vi "WS1021 CP Setting.vi"(4 "Manual Setting":i32(ring) items=["CP OFF", "CP ON", "OTP OFF", "CP 24V", "CP 26V", "CP 28V", "CP 30V", "CP 31V", "CP 32V", "CP 33V", "CP 34V", "CP 35V", "CP 36V", "CP 37V", "CP 38V", "CP 39V", "CP 40V", "CP 41V", "CP 42V", "CP 43V", "CP 44V", "CP 45V", "CP 46V", "CP 47V", "CP 48V", "CP 49V", "CP 50V", "CP 51V", "CP 52V", "CP 53V", "CP 54V", "CP 56V", "CP 58V", "CP 60V", "CP 62V"], 6 "FPGA":T1, 8 "Error In":errorcluster) -> (0 "Error Out":errorcluster, 3 "CP Select":string)   [LabVIEW 2017]
uses:
  WS_VCAP Driver 039/Source/WSVCAP Shell/Type Defs/WSVCAP SHL FPGA Enum.ctl
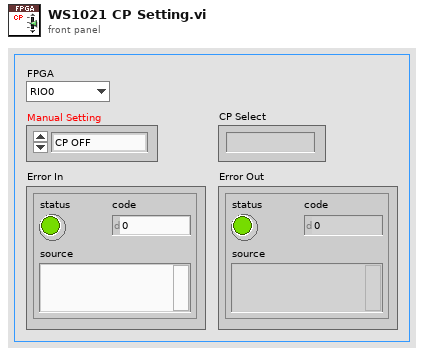
[diagram p1: front panel]
types:
  T1 = typedef "WSVCAP SHL FPGA Enum.ctl" = enum16{"RIO0", "RIO1"}
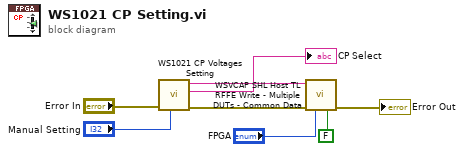
[diagram p0: block diagram]
diagram:
  n1 = call "WS1021 CP Voltages Setting.vi"("Select CPV"="Manual Setting", "Error In"="Error In") -> ("Error Out"=w8:errorcluster, "CP Select"=→"CP Select":string, "Cmd Send out"=w7:string)  [unwired: 4 in, 3 out]
  n2 = call "WSVCAP SHL Host TL RFFE Write - Multiple DUTs - Common Data.vi"("Data Out"=w7, "error in"=w8, "FPGA"="FPGA", "Log (T)"=FALSE) -> ("error out"=→"Error Out":errorcluster)  [unwired: 11 in]
